vi "DB_Selectv2.vi"(8 "error in (no error)":errorcluster, 11 "SQLite Connection in":refnum<class "Connection.lvclass">) -> (0 "error out":errorcluster, 2 "Result Set":string[][](table) caption="Result Set (from first statement with results)", 3 "SQLite Connection":refnum<class "Connection.lvclass">)   [LabVIEW 2020]
uses:
  <vilib>/drjdpowell/SQLite Library/SQL Connection/Connection.lvclass
  <vilib>/drjdpowell/SQLite Library/SQL Connection/Execute SQL.vi
  <vilib>/drjdpowell/SQLite Library/SQLite.lvlib
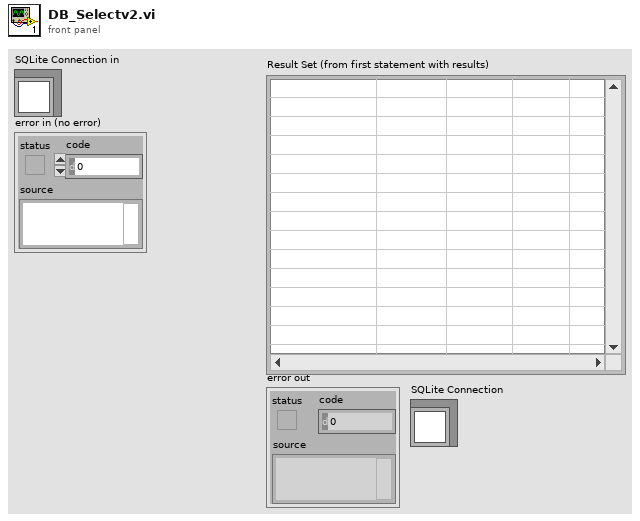
[diagram p1: front panel]
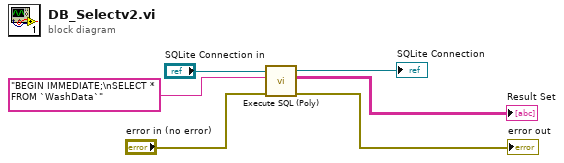
[diagram p0: block diagram]
diagram:
  n1 = call-poly <vilib>:"Execute SQL (Poly).vi"("error in (no error)"="error in (no error)", "SQL"="BEGIN IMMEDIATE;\nSELECT * FROM `WashData`", "SQLite Connection in"="SQLite Connection in") -> ("error out"=→"error out":errorcluster, "Result Set"=→"Result Set":string[][], "SQLite Connection"=→"SQLite Connection":refnum<class "Connection.lvclass">)  [unwired: 5 in, 1 out]
